vi "Plot Signal.vi"(8 "error in (no error)":errorcluster, 9 "XY Graph":refnum<vi>, 10 "Signal Name":string(combo), 11 "Signal Analysis in":refnum<class "Signal Analysis.lvclass">) -> (0 "error out":errorcluster, 3 "Signal Analysis out":refnum<class "Signal Analysis.lvclass">)   [LabVIEW 2023, in "Data Analysis.lvlib" / "Signal Analysis.lvlib" / "Signal Analysis.lvclass"]
uses:
  Signal Analysis.lvclass
  Signal Analysis.lvclass/Signal Analysis.ctl
  HardwareAbstractionLayer_LVOOP/Database/Database.lvclass
panel:
  out "XY Graph":cluster{dbl[], dbl[]}[](graph) caption="XY Graph - Dark"
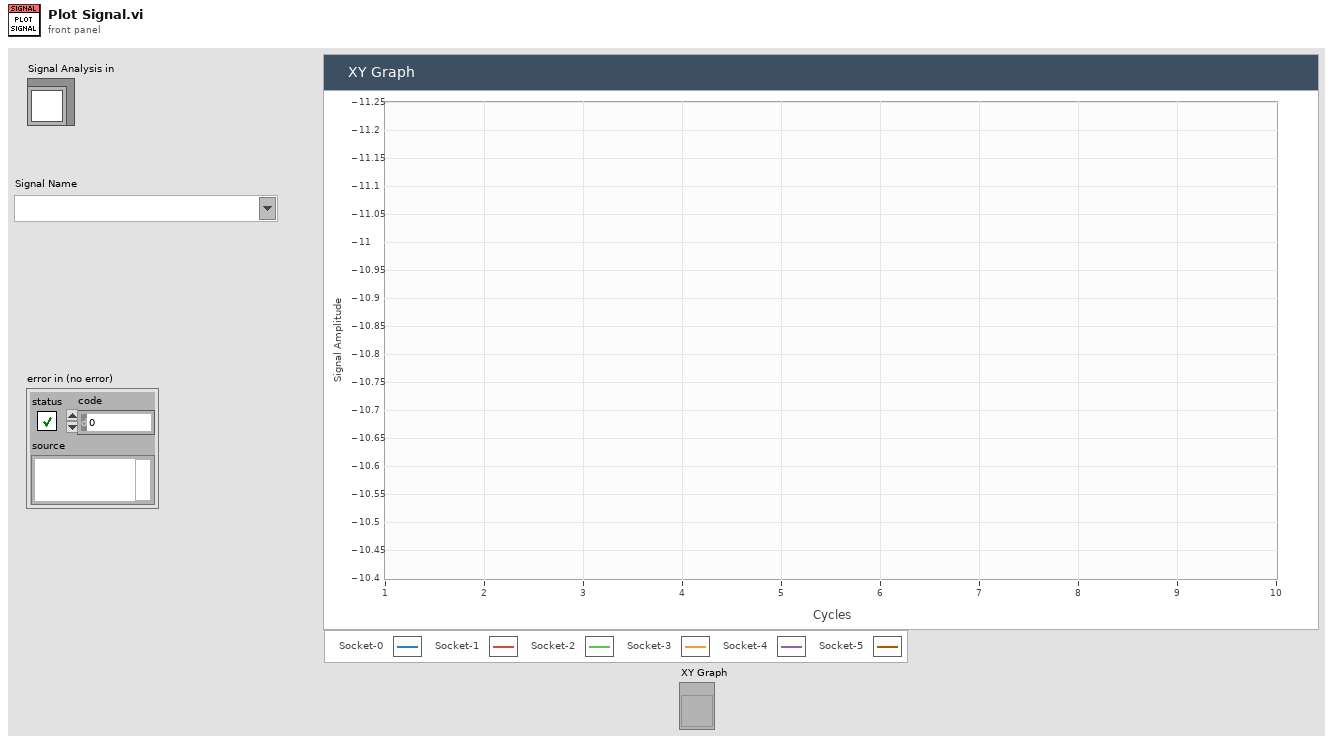
[diagram p1: front panel]
types:
  T1 = cluster{"Socket 0":bool, "Socket 1":bool, "Socket 2":bool, "Socket 3":bool, "Socket 4":bool, "Socket 5":bool}
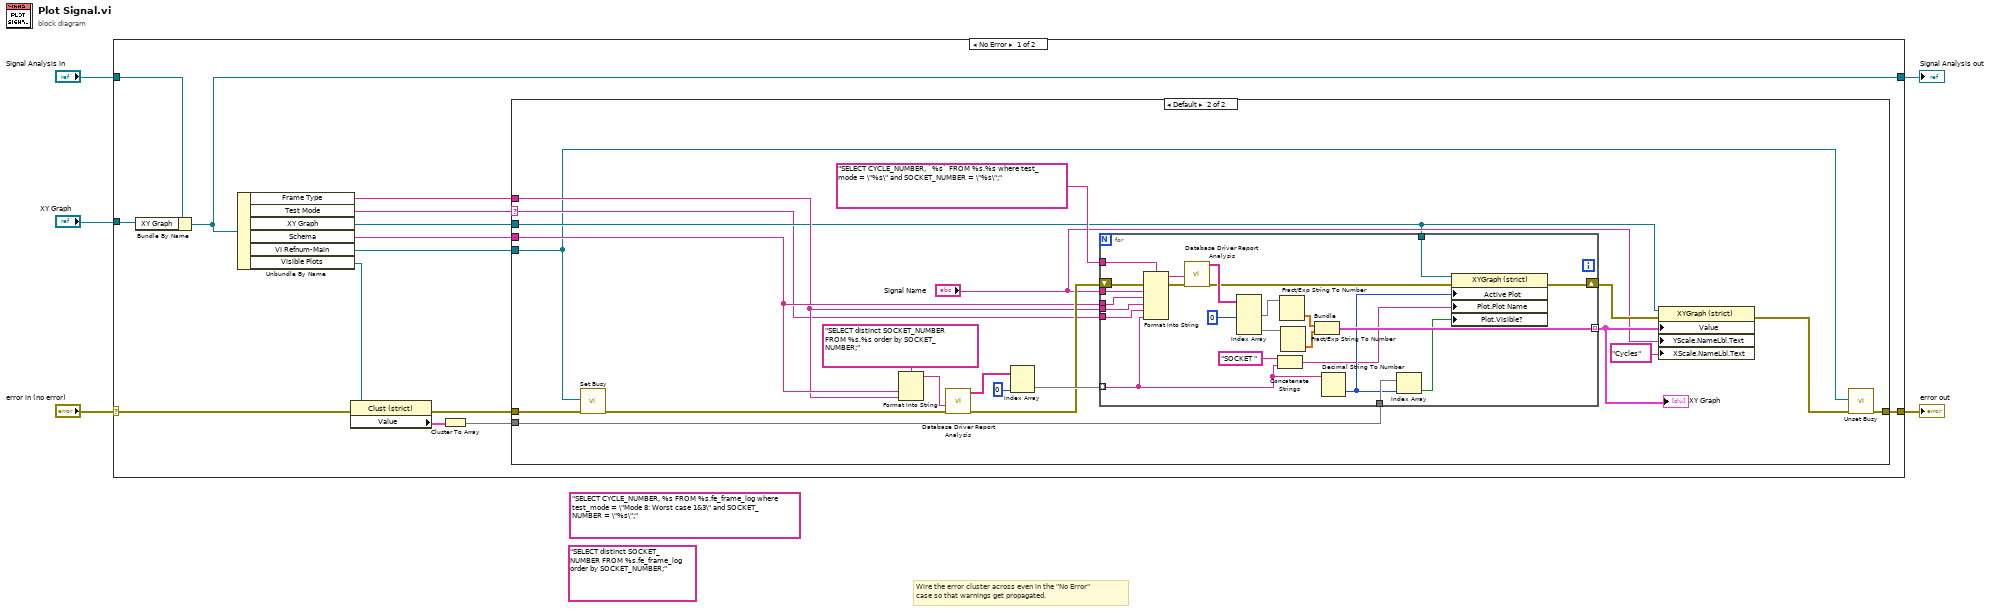
[diagram p0: block diagram]
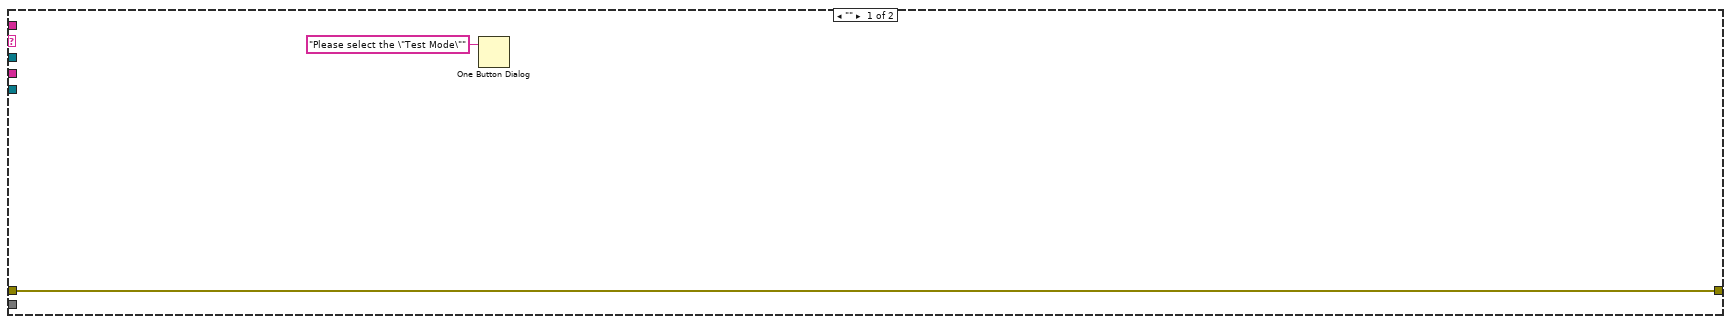
[diagram p2: hidden frame]
diagram:
  (unwired) "SELECT distinct SOCKET_NUMBER FROM %s.fe_frame_log order by SOCKET_NUMBER;"
  (unwired) "SELECT CYCLE_NUMBER, %s FROM %s.fe_frame_log where test_mode = \"Mode 8: Worst case 1&3\" and SOCKET_NUMBER = \"%s\";"
  # "Wire the error cluster across even in the \"No Error\"\ncase so that warnings get propagated."
  n1 = case shown="No Error" "error in (no error)" {
    selector: "error in (no error)" -> [w9 w68]
    tunnel: [w11 w68] -> w4
    tunnel: [w12 w67] -> w2
    tunnel: "Signal Analysis in" -> [w17 w67]
    tunnel: "XY Graph" -> [w16 _]
    frame No Error {
      n2 = Bundle By Name(cluster=w17, "XY Graph"=w16) -> (w12:refnum<class "Signal Analysis.lvclass">)
      n3 = Unbundle By Name(w12) -> ("Frame Type"=w18:string, "Test Mode"=w14:string, "XY Graph"=w15:refnum<vi>, "Schema"=w19:string, "VI Refnum-Main"=w13:refnum<vi>, "Visible Plots"=w10:refnum<vi>)
      n4 = property class="Clust (strict)"(reference=w10, error in=w9) -> (error out=w8:errorcluster, "Value"=w7:T1)  [unwired: 1 out]
      n5 = Cluster To Array(cluster=w7) -> (array=w6:bool[])
      n6 = case shown="Default" w14 {
        selector: w14 -> [_ w28]
        tunnel: w19 -> [_ w36]
        tunnel: w18 -> [_ w32]
        tunnel: w15 -> [_ w29]
        tunnel: w8 -> [w21 w27]
        tunnel: w13 -> [_ w23]
        tunnel: [w21 w24] -> w11
        tunnel: w6 -> [_ w22]
        frame "" {
          n7 = One Button Dialog(message="Please select the \"Test Mode\"") -> ()  [unwired: 1 in, 1 out]
        }
        frame Default {
          n8 = call <vilib>:"Set Busy.vi"("error in (no error)"=w27, "VI reference (current VI)"=w23) -> ("error out"=w26:errorcluster)  [unwired: 8 in, 1 out]
          n9 = Format Into String(format string="SELECT distinct SOCKET_NUMBER FROM %s.%s order by SOCKET_NUMBER;", w36, w32) -> (resulting string=w41:string)  [unwired: 2 in, 1 out]
          n10 = call "Database Driver Report Analysis.vi"("error in"=w26, "SQL query"=w41) -> ("error out"=w37:errorcluster, "data"=w40:string[][])  [unwired: 6 in, 2 out]
          n11 = Index Array(array=w40, index (col)=0 ("disabled index (col)")) -> (element=w39:string[])  [unwired: 1 in]
          n12 = for {
            tunnel: w39 -> [w43] mode=indexing
            tunnel: "SELECT CYCLE_NUMBER, `%s` FROM %s.%s where test_mode = \"%s\" and SOCKET_NUMBER = \"%s\";" -> [w66]
            tunnel: "Signal Name" -> [w65]
            tunnel: w36 -> [w64]
            shift-right: [w51] -> w34
            shift-left: w37 -> [w61]
            tunnel: [w54] -> w35 mode=indexing
            tunnel: w29 -> [w50]
            tunnel: w32 -> [w49]
            tunnel: w28 -> [w48]
            tunnel: w22 -> [w47]
            n13 = Format Into String(format string=w66, error in=w61, w65, w64, w49, w48, w43) -> (resulting string=w63:string, error out=w62:errorcluster)  [unwired: 1 in]
            n14 = call "Database Driver Report Analysis.vi"("error in"=w62, "SQL query"=w63) -> ("error out"=w53:errorcluster, "data"=w60:string[][])  [unwired: 6 in, 2 out]
            n15 = Index Array(array=w60, index (col) #1=0 ("disabled index (col)")) -> (element #1=w58:string[], element #2=w56:string[])  [unwired: 3 in]
            n16 = Concatenate Strings("SOCKET " ("string"), w43) -> (w44:string)
            n17 = Fract/Exp String To Number(string=w58) -> (number=w57:dbl[])  [unwired: 3 in, 1 out]
            n18 = Fract/Exp String To Number(string=w56) -> (number=w55:dbl[])  [unwired: 3 in, 1 out]
            n19 = Bundle(w57, w55) -> (w54:cluster{dbl[], dbl[]})  [unwired: 1 in]
            n20 = Decimal String To Number(string=w43) -> (number=w46:i32)  [unwired: 2 in, 1 out]
            n21 = Index Array(array=w47, index=w46) -> (element=w45:bool)
            n22 = property class="XYGraph (strict)"(reference=w50, error in=w53, "Active Plot"=w46, "Plot.Plot Name"=w44, "Plot.Visible?"=w45) -> (error out=w51:errorcluster)  [unwired: 1 out]
          }
          "XY Graph" <- w35
          n23 = property class="XYGraph (strict)"(reference=w29, error in=w34, "Value"=w35, "YScale.NameLbl.Text"="Signal Name", "XScale.NameLbl.Text"="Cycles" ("X Scale.Name Label.Text")) -> (error out=w25:errorcluster)  [unwired: 1 out]
          n24 = call <vilib>:"Unset Busy.vi"("error in (no error)"=w25, "VI reference (current VI)"=w23) -> ("error out"=w24:errorcluster)  [unwired: 9 in]
        }
      }
    }
    frame Error {
    }
  }
  "error out" <- w4
  "Signal Analysis out" <- w2
